vi "RIGOL DG4000 Series Modulated Waveform.vi"() -> ()   [LabVIEW 2012]
doc: "This example shows how to generate a modulated waveform."
uses:
  <instrlib>/RIGOL DG4000 Series/Public/Configure/Configure Standard Waveform(Sine).vi
  <instrlib>/RIGOL DG4000 Series/Public/Configure/Modulation/Configure Modulation(Amplitude).vi
  <instrlib>/RIGOL DG4000 Series/RIGOL DG4000 Series.lvlib
panel:
  in  "Modulation Depth (100 %)":dbl=100.0
  in  "Modulation Frequency (100 Hz)":dbl=100.0
  in  "Modulation Waveform (0: Sinusoid)":i32(ring) items=["Sinusoid", "Square", "Triangle", "Ramp", "Nramp", "Noise", "User"]
  in  "AM Source (0: Internal)":i32(ring) items=["Internal", "External"]
  in  "Output Channel (1: Channel 1)":i32(ring)=1 items=["Channel 1"=1, "Channel 2"=2]
  in  "DC Offset (0.00 V)":dbl
  in  "Frequency (1000 Hz)":dbl=1000.0
  in  "Amplitude (0.1 Vpp)":dbl=0.1
  in  "VISA resource name":refnum<visa-resource-name>
  # "(c) 2012 National Instruments.  ALL RIGHTS RESERVED."
  # "Carrier Settings"
  # "Modulation Settings"
  # "To change the carrier waveform shape, select the corressponding poly-subVI of the Configure Standard Waveform.vi. It is Sine by default."
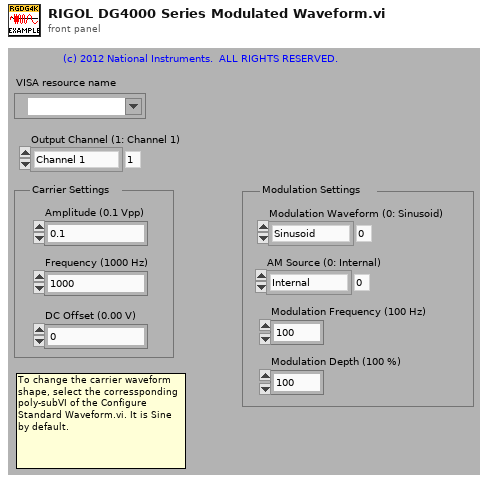
[diagram p1: front panel]
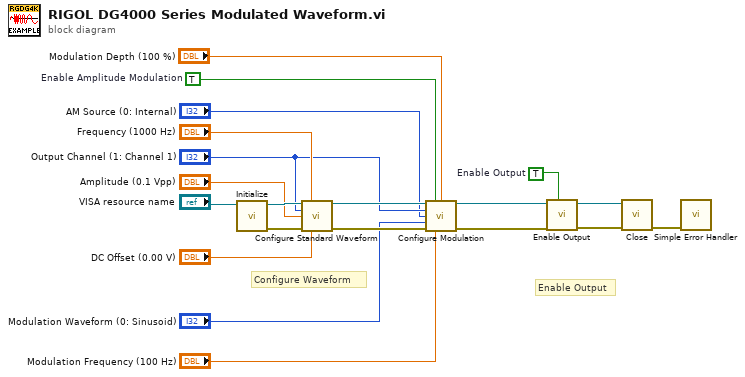
[diagram p0: block diagram]
diagram:
  w6 = TRUE  # Enable Amplitude Modulation
  w11 = TRUE  # Enable Output
  # "Enable Output"
  # "Configure Waveform"
  n1 = call <instrlib>:"Initialize.vi"("VISA resource name"="VISA resource name") -> ("error out"=w18:errorcluster, "VISA resource name out"=w19:refnum<visa-resource-name>)  [unwired: 4 in, 5 out]
  n2 = call-poly <instrlib>:"Configure Standard Waveform.vi"("VISA resource name"=w19, "Frequency (1000 Hz)"="Frequency (1000 Hz)", "Output Channel (1: Channel 1)"="Output Channel (1: Channel 1)", "Amplitude (5 Vpp)"="Amplitude (0.1 Vpp)", "error in (no error)"=w18, "Offset (0)"="DC Offset (0.00 V)") -> ("VISA resource name out"=w10:refnum<visa-resource-name>, "error out"=w8:errorcluster)  [unwired: 2 in, 6 out]
  n3 = call-poly <instrlib>:"Configure Modulation.vi"("VISA resource name"=w10, "Enable Amplitude Modulation (F: Disable)"=w6, "Modulation Depth (100 %)"="Modulation Depth (100 %)", "Channel (1: Channel 1)"="Output Channel (1: Channel 1)", "AM Source (0: Internal)"="AM Source (0: Internal)", "Modulation Waveform (0: Sinusoid)"="Modulation Waveform (0: Sinusoid)", "error in (no error)"=w8, "Modulation Frequency (100 Hz)"="Modulation Frequency (100 Hz)") -> ("VISA resource name out"=w9:refnum<visa-resource-name>, "error out"=w7:errorcluster)  [unwired: 6 out]
  n4 = call <instrlib>:"Enable Output.vi"("Enable Output (T: Enable)"=w11, "error in (no error)"=w7, "VISA resource name"=w9) -> ("error out"=w13:errorcluster, "VISA resource name out"=w14:refnum<visa-resource-name>)  [unwired: 1 in, 6 out]
  n5 = call <instrlib>:"Close.vi"("error in (no error)"=w13, "VISA resource name"=w14) -> ("error out"=w15:errorcluster)  [unwired: 9 out]
  n6 = call <vilib>:"Simple Error Handler.vi"("error in (no error)"=w15) -> ()  [unwired: 1 in, 8 out]
